vi "Import SQL.vi"(8 "error in (no error)":errorcluster, 10 "Import Data":T1, 11 "Import Export SQL in":refnum<class "Import Export SQL.lvclass">) -> (0 "error out":errorcluster, 3 "Import Export SQL out":refnum<class "Import Export SQL.lvclass">)   [LabVIEW 2023, in "Data Analysis.lvlib" / "Import Export SQL.lvlib" / "Import Export SQL.lvclass"]
uses:
  Import Export SQL.lvclass
  <vilib>/Utility/sysdir.llb/System Directory Type.ctl
  Import Export SQL.lvclass/Import Export SQL.ctl
  259c5827-dcf7-4c29-9ce9-e7b34ea6383a.vi
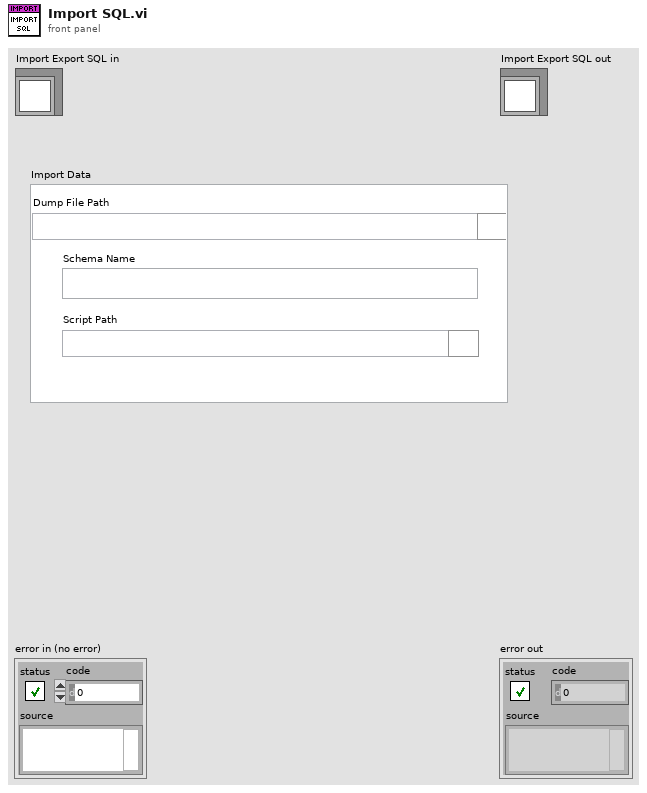
[diagram p1: front panel]
types:
  T1 = cluster{"Schema Name":string, "Dump File Path":path, "Script Path":path}
  T2 = typedef "System Directory Type.ctl" = i32
  T3 = enum16{"open", "replace", "create", "open or create", "replace or create", "replace or create with confirmation"}
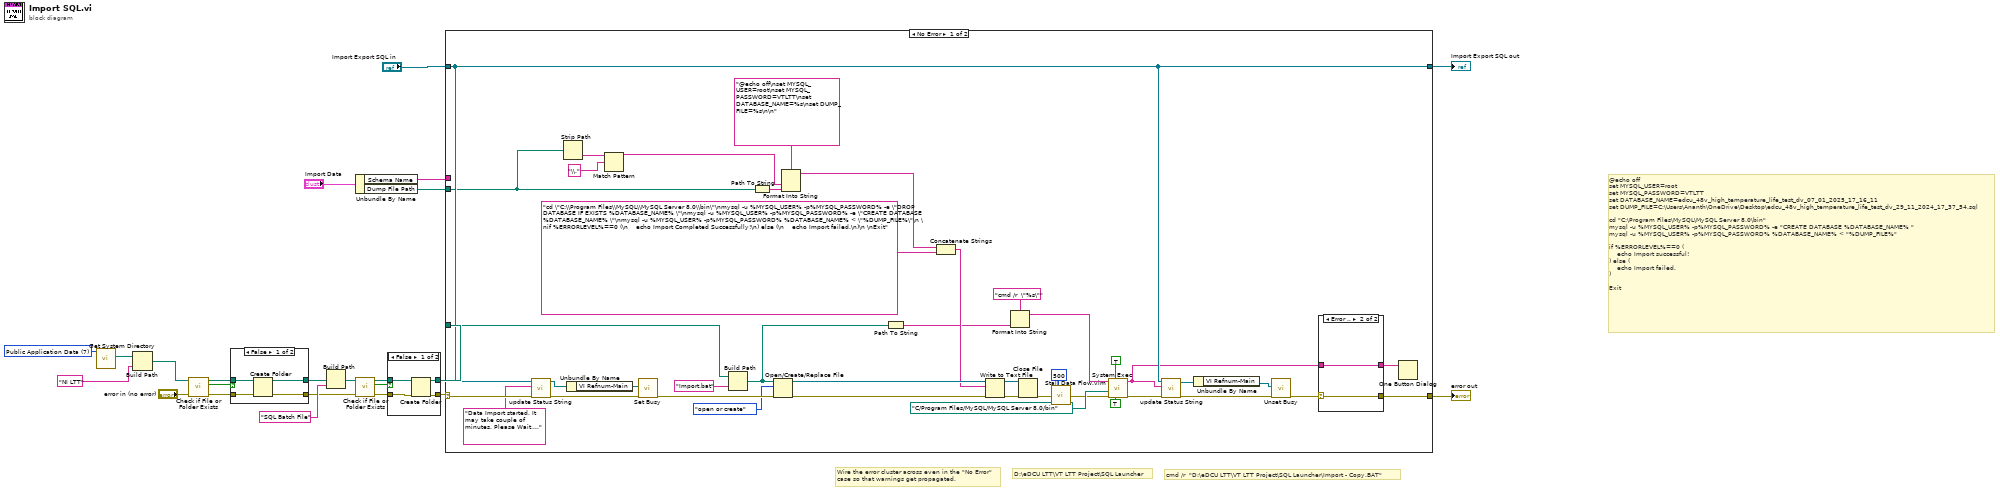
[diagram p0: block diagram]
diagram:
  w8 = T2 7 items=["User Home"=0, "User Desktop"=1, "User Documents"=2, "User Application Data"=3, "User Preferences"=4, "User Temporary"=5, "Public Documents"=6, "Public Application Data"=7, "Public Preferences"=8, "Public Cache"=13, "System Core Libraries"=9, "System Installed Libraries"=10, "Application Files"=11, "Boot Volume Root"=12] ("system directory type")
  # "@echo off\nset MYSQL_USER=root\nset MYSQL_PASSWORD=VTLTT\nset DATABASE_NAME=edcu_48v_high_temperature_life_test_dv_07_01_2025_17_16_11\nset DUMP_FILE=C:\\Users\\Ananth\\OneDrive\\Desktop\\edcu_48v_high_temperature_life_test_dv_29_11_2024_17_37_54.sql\n\ncd \"C:\\Program Files\\MySQL\\MySQL Server 8.0\\bin\"\nmysql -u %MYSQL_USER% -p%MYSQL_PASSWORD% -e \"CREATE DATABASE %DATABASE_NAME% \"\nmysql -u %MYSQL_USER% -p%MYSQL_PASSWORD% %DATABASE_NAME% < \"%DUMP_FILE%\"\n \nif %ERRORLEVEL%==0 (\n    echo Import successful!\n) else (\n    echo Import failed.\n)\n \nExit"
  # "Wire the error cluster across even in the \"No Error\"\ncase so that warnings get propagated."
  # "D:\\eDCU LTT\\VT LTT Project\\SQL Launcher"
  # "cmd /r  \"D:\\eDCU LTT\\VT LTT Project\\SQL Launcher\\Import - Copy.BAT\""
  n1 = call <vilib>:"Get System Directory.vi"("system directory type"=w8) -> ("system directory"=w9:path)  [unwired: 10 in]
  n2 = Build Path(base path=w9, name or relative path="NI LTT") -> (appended path=w4:path)
  n3 = call <vilib>:"Check if File or Folder Exists.vi"("error in (no error)"="error in (no error)", "path"=w4) -> ("error out"=w5:errorcluster, "file or folder exists?"=w6:bool, "dup path"=w7:path)  [unwired: 7 in]
  n4 = case shown="False" w6 {
    tunnel: w5 -> [w27 w29]
    tunnel: [w26 w29] -> w2
    tunnel: w7 -> [w25 w28]
    tunnel: [w24 w28] -> w3
    frame False {
      n5 = Create Folder(path (use dialog)=w25, error in=w27) -> (created path=w24:path, error out=w26:errorcluster)  [unwired: 1 in, 1 out]
    }
    frame True {
    }
  }
  n6 = Build Path(base path=w3, name or relative path="SQL Batch File") -> (appended path=w15:path)
  n7 = Unbundle By Name("Import Data") -> ("Schema Name"=w19:string, "Dump File Path"=w18:path)
  n8 = call <vilib>:"Check if File or Folder Exists.vi"("error in (no error)"=w2, "path"=w15) -> ("error out"=w16:errorcluster, "file or folder exists?"=w14:bool, "dup path"=w13:path)  [unwired: 7 in]
  n9 = case shown="False" w14 {
    tunnel: w16 -> [w33 w35]
    tunnel: [w32 w35] -> w12
    tunnel: w13 -> [w31 w34]
    tunnel: [w30 w34] -> w11
    frame False {
      n10 = Create Folder(path (use dialog)=w31, error in=w33) -> (created path=w30:path, error out=w32:errorcluster)  [unwired: 1 in, 1 out]
    }
    frame True {
    }
  }
  n11 = case shown="No Error" w12 {
    selector: w12 -> [w47 w82]
    tunnel: [w55 w82] -> w23
    tunnel: [w43 w81] -> w21
    tunnel: "Import Export SQL in" -> [w43 w81]
    tunnel: w19 -> [_ _]
    tunnel: w11 -> [w61 _]
    tunnel: w18 -> [w37 _]
    frame No Error {
      n12 = call "update Status String.vi"("error in (no error)"=w47, "Data to Append"="Data Import started, It may take couple of  minutes. Please Wait....", "Import Export SQL in"=w43) -> ("error out"=w46:errorcluster, "Import Export SQL out"=w48:refnum<class "Import Export SQL.lvclass">)  [unwired: 7 in]
      n13 = Strip Path(path=w37) -> (name=w39:string)  [unwired: 1 out]
      n14 = Unbundle By Name(w48) -> ("VI Refnum-Main"=w59:refnum<vi>)
      n15 = Match Pattern(string=w39, regular expression="\\.") -> (before substring=w36:string)  [unwired: 1 in, 3 out]
      n16 = call <vilib>:"Set Busy.vi"("error in (no error)"=w46, "VI reference (current VI)"=w59) -> ("error out"=w58:errorcluster)  [unwired: 8 in, 1 out]
      n17 = Build Path(base path=w61, name or relative path="Import.bat") -> (appended path=w53:path)
      n18 = Path To String(path=w37) -> (string=w68:string)
      n19 = Open/Create/Replace File(file path (use dialog)=w53, error in=w58, operation (0:open)=T3."open or create") -> (refnum out=w76:refnum<file>, error out=w75:errorcluster)  [unwired: 3 in, 1 out]
      n20 = Format Into String(format string="@echo off\nset MYSQL_USER=root\nset MYSQL_PASSWORD=VTLTT\nset DATABASE_NAME=%s\nset DUMP_FILE=%s\n\n", w36, w68) -> (resulting string=w72:string)  [unwired: 2 in, 1 out]
      n21 = Path To String(path=w53) -> (string=w60:string)
      n22 = Concatenate Strings(w72, "cd \"C:\\Program Files\\MySQL\\MySQL Server 8.0\\bin\"\nmysql -u %MYSQL_USER% -p%MYSQL_PASSWORD% -e \"DROP DATABASE IF EXISTS %DATABASE_NAME% \"\nmysql -u %MYSQL_USER% -p%MYSQL_PASSWORD% -e \"CREATE DATABASE %DATABASE_NAME% \"\nmysql -u %MYSQL_USER% -p%MYSQL_PASSWORD% %DATABASE_NAME% < \"%DUMP_FILE%\"\n \nif %ERRORLEVEL%==0 (\n    echo Import Completed Successfully!\n) else (\n    echo Import failed.\n)\n \nExit") -> (w70:string)
      n23 = Write to Text File(file (use dialog)=w76, text=w70, error in=w75) -> (refnum out=w73:refnum<file>, error out=w74:errorcluster)  [unwired: 1 in, 1 out]
      n24 = Format Into String(format string="cmd /r  \"%s\"" ("command line"), w60) -> (resulting string=w62:string)  [unwired: 2 in, 1 out]
      n25 = Close File(refnum=w73, error in=w74) -> (error out=w67:errorcluster)  [unwired: 1 out]
      n26 = call "Stall Data Flow.vim"("value in"=w67, "milliseconds to wait"=u32 500) -> ("value out"=w49:errorcluster)  [unwired: 1 out]
      n27 = call <vilib>:"System Exec.vi"("run minimized? (F)"=TRUE, "wait until completion? (T)"=TRUE, "error in (no error)"=w49, "working directory"=path "C:/Program Files/MySQL/MySQL Server 8.0/bin", "command line"=w62) -> ("error out"=w45:errorcluster, "standard output"=w41:string)  [unwired: 3 in, 2 out]
      n28 = call "update Status String.vi"("error in (no error)"=w45, "Data to Append"=w41, "Import Export SQL in"=w43) -> ("error out"=w44:errorcluster, "Import Export SQL out"=w42:refnum<class "Import Export SQL.lvclass">)  [unwired: 7 in]
      n29 = Unbundle By Name(w42) -> ("VI Refnum-Main"=w57:refnum<vi>)
      n30 = call <vilib>:"Unset Busy.vi"("error in (no error)"=w44, "VI reference (current VI)"=w57) -> ("error out"=w56:errorcluster)  [unwired: 9 in]
      n31 = case shown="Error .." w56 {
        selector: w56 -> [w78 w80]
        tunnel: [w78 w80] -> w55
        tunnel: w41 -> [w77 w79]
        tunnel: [w77 w79] -> w54
        frame No Error {
        }
        frame Error {
        }
      }
      n32 = One Button Dialog(message=w54) -> ()  [unwired: 1 in, 1 out]
    }
    frame Error {
    }
  }
  "error out" <- w23
  "Import Export SQL out" <- w21
